vi "Get Root Path.vi"() -> (0 "root path":path)   [LabVIEW 2013]
doc: "Returns path to the root of the project. It is project root folder in development version and it is compiled application root foler if it is runtime application."
uses:
  varilib/varilib.lvlib
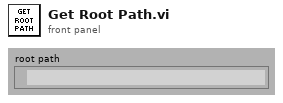
[diagram p1: front panel]
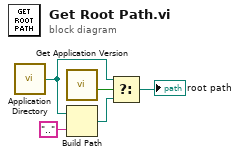
[diagram p0: block diagram]
diagram:
  n1 = call <vilib>:"Application Directory.vi"() -> ("Application Directory"=w1:path)
  n2 = call "Get Application Version.vi"() -> ("run time system"=w2:bool)  [unwired: 8 in, 3 out]
  n3 = Build Path(base path=w1, name or relative path="..") -> (appended path=w3:path)
  n4 = Select(t=w1, s=w2, f=w3) -> (s? t:f=→"root path":path)
